vi "test Search 2D Array for Element Inorrect.vi"(8 "error in (no error)":errorcluster, 11 "TestCase in":refnum<class "Utility VIs tests.lvclass">) -> (0 "error out":errorcluster, 3 "TestCase out":refnum<class "Utility VIs tests.lvclass">)   [LabVIEW 2014, in "Utility VIs tests.lvclass"]
uses:
  Utility VIs tests.lvclass
  <vilib>/addons/_JKI Toolkits/VI Tester/TestCase.llb/TestCase.lvclass
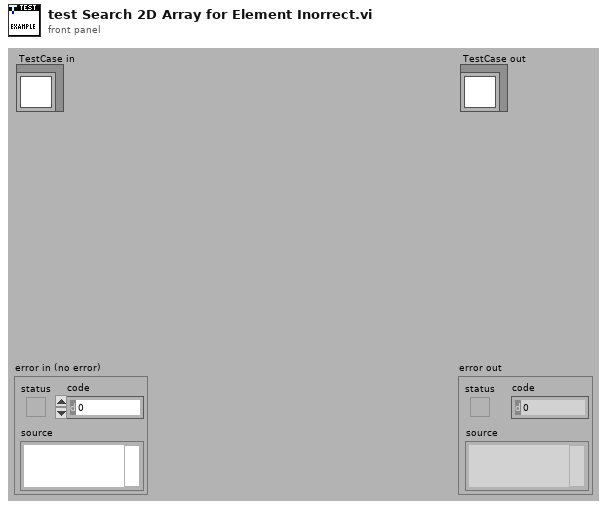
[diagram p1: front panel]
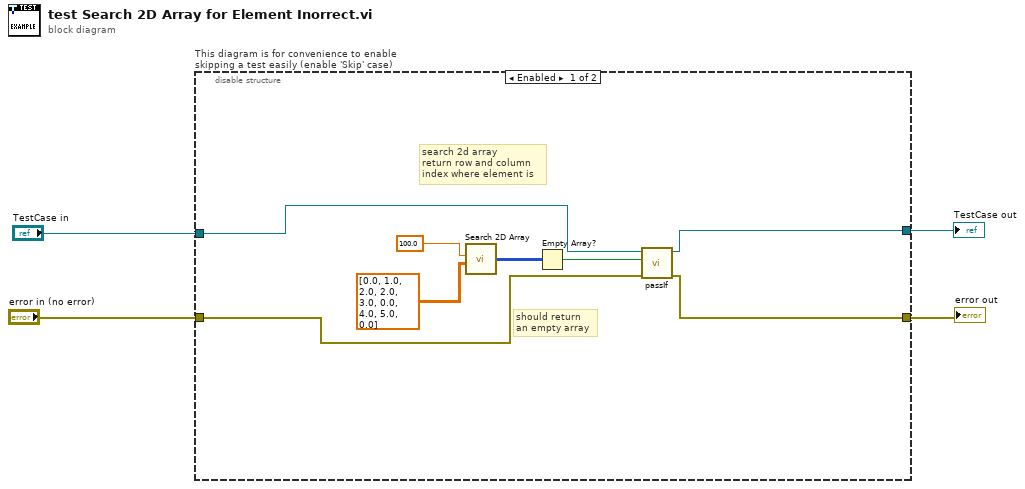
[diagram p0: block diagram]
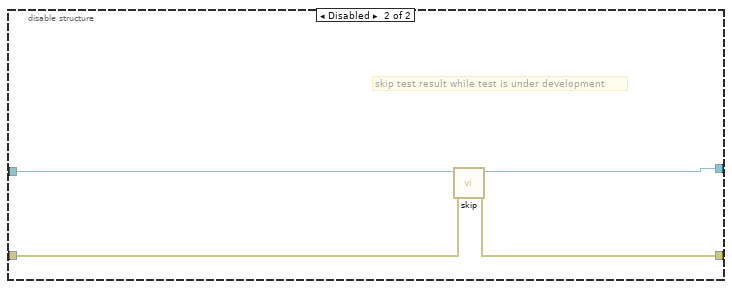
[diagram p2: hidden frame]
diagram:
  n1 = disable-structure "This diagram is for convenience to enable skipping a test easily (enable 'Skip' case)" shown="Enabled" {
    disable-tunnel: "TestCase in" -> [w6 w16]
    disable-tunnel: [w8 w14] -> w1
    disable-tunnel: [w7 w15] -> w3
    disable-tunnel: "error in (no error)" -> [w5 w13]
    frame Enabled {
      # "should return\nan empty array"
      # "search 2d array\nreturn row and column\nindex where element is"
      n2 = call "Search 2D Array.vi"("Element"=100.0, "Array"=dbl[][] [[0.0, 1.0, 2.0], [2.0, 3.0, 0.0], [4.0, 5.0, 0.0]]) -> ("Locations"=w10:i32[][])  [unwired: 5 in]
      n3 = Empty Array?(array=w10) -> (empty?=w9:bool)
      n4 = call-dynamic "passIf.vi"("error in (no error)"=w5, "pass"=w9, "TestCase in"=w6) -> ("error out"=w7:errorcluster, "TestCase out"=w8:refnum<class "Utility VIs tests.lvclass">)  [unwired: 7 in]
    }
    frame Disabled {
      # "skip test result while test is under development"
      n5 = call <vilib>:"skip.vi"("error in (no error)"=w13, "TestCase in"=w16) -> ("error out"=w15:errorcluster, "TestCase out"=w14:refnum<class "Utility VIs tests.lvclass">)  [unwired: 8 in]
    }
  }
  "error out" <- w3
  "TestCase out" <- w1
